vi "Version_4.9_8_on-chip_valves_for25ulSyringe_withModfied_Plunging.vi"() -> ()   [LabVIEW 2020] (continued)
                                n1270 = call "GoToAbsolutePosition(SubVI).vi"("Absolute Volume Position in Syringe (in ul)"=0.0 ("Volume to be Dispensed"), "Volume of Syringe"=w1733, "Resolution of Pumping"=w1732, "Flow Rate (ul/min)"=w1724, "VISA Refnum in"=w1734) -> ()  [unwired: 6 in, 1 out]
                                n1271 = local read "VISA Refnum in\nfor Valve"() -> (w1726:refnum<visa-resource-name>)
                                n1272 = local read "External Valve \nOPEN"() -> (w1725:string)
                                n1273 = local write "Valve V2 Open"(TRUE ("Valve V2 Open")) -> ()
                                n1274 = local write "Valve V1 Open"(FALSE ("Valve V1 Open")) -> ()
                                n1275 = local write "Valve V4 Open"(FALSE ("Valve V4 Open")) -> ()
                                n1276 = local write "Valve V3 Open"(TRUE ("Valve V3 Open")) -> ()
                                n1277 = call "PortChanger_Valve (SubVI).vi"("Port Number"=w1725, "VISA Refnum in"=w1726) -> ()  [unwired: 10 in]
                                }
                                frame #5 {
                                n1278 = local read "VISA Refnum in\nfor Pump"() -> (w1735:refnum<visa-resource-name>)
                                n1279 = call "ProcessCompletionWaiter (SubVI).vi"("VISA Refnum in"=w1735) -> ()  [unwired: 11 in]
                                }
                                frame #6 {
                                # "Change the port back to Buffer-C1"
                                n1280 = local read "VISA Refnum in\nfor Pump"() -> (w1737:refnum<visa-resource-name>)
                                n1281 = local read "Port for \nC1-Equilibriation"() -> (w1736:string)
                                n1282 = call "PortChanger (SubVI).vi"("Port Number"=w1736, "VISA Refnum in"=w1737) -> ()  [unwired: 10 in]
                                }
                                frame #7 {
                                n1283 = local read "VISA Refnum in\nfor Pump"() -> (w1738:refnum<visa-resource-name>)
                                n1284 = call "ProcessCompletionWaiter (SubVI).vi"("VISA Refnum in"=w1738) -> ()  [unwired: 11 in]
                                }
                              }
                            }
                          }
                          frame #4 {
                            # "Washes the SEC column"
                            n1285 = local read "Apparent Volume\nof Syringe"() -> (w1741:dbl)
                            n1286 = local read "c"() -> (w1742:dbl)
                            n1287 = Quotient & Remainder(x=w1742, y=w1741) -> (x-y*floor(x/y)=w1740:dbl, floor(x/y)=w1739:dbl)
                            n1288 = for {
                              N: w1739 -> [_]
                              n1289 = stacked-sequence {
                                frame #0 {
                                n1290 = local read "Buffer-A2 Pumping\nResolution"() -> (w1745:T2)
                                n1291 = local read "VISA Refnum in\nfor Pump"() -> (w1747:refnum<visa-resource-name>)
                                n1292 = local read "Apparent Volume\nof Syringe"() -> (w1743:dbl)
                                n1293 = local read "Volume of Syringe"() -> (w1746:dbl)
                                n1294 = call "RPickUp(SubVI).vi"("Volume to be picked up"=w1743, "Volume of Syringe"=w1746, "Resolution of PickUP"=w1745, "PickUp Flow Rate (ul/min)"=150.0, "VISA Refnum in"=w1747) -> ()  [unwired: 6 in, 1 out]
                                }
                                frame #1 {
                                n1295 = local read "Stopper that ends \nthe main loops"() -> (w1748:bool)
                                n1296 = local read "VISA Refnum in\nfor Pump"() -> (w1749:refnum<visa-resource-name>)
                                n1297 = case shown="True" w1748 {
                                frame False {
                                }
                                frame True {
                                n1298 = local read "VISA Refnum in\nfor Pump"() -> (w1750:refnum<visa-resource-name>)
                                n1299 = call "HardStopCurrentProcess (SubVI).vi"("VISA Refnum in"=w1750) -> ()  [unwired: 11 in]
                                }
                                }
                                n1300 = call "ProcessCompletionWaiter (SubVI).vi"("VISA Refnum in"=w1749) -> ()  [unwired: 11 in]
                                }
                                frame #2 {
                                # "Switch to Port-10"
                                # "Port-10 of the pump is conncted to column-2 of chip"
                                n1301 = local read "VISA Refnum in\nfor Pump"() -> (w1752:refnum<visa-resource-name>)
                                n1302 = call "PortChanger (SubVI).vi"("Port Number"="10", "VISA Refnum in"=w1752) -> ()  [unwired: 10 in]
                                }
                                frame #3 {
                                n1303 = local read "Stopper that ends \nthe main loops"() -> (w1753:bool)
                                n1304 = local read "VISA Refnum in\nfor Pump"() -> (w1754:refnum<visa-resource-name>)
                                n1305 = case shown="True" w1753 {
                                frame False {
                                }
                                frame True {
                                n1306 = local read "VISA Refnum in\nfor Pump"() -> (w1755:refnum<visa-resource-name>)
                                n1307 = call "HardStopCurrentProcess (SubVI).vi"("VISA Refnum in"=w1755) -> ()  [unwired: 11 in]
                                }
                                }
                                n1308 = call "ProcessCompletionWaiter (SubVI).vi"("VISA Refnum in"=w1754) -> ()  [unwired: 11 in]
                                }
                                frame #4 {
                                # "Keeps the AMF valve after column-1 open and valve after column-2 closed"
                                n1309 = local read "Buffer-A2 Pumping\nResolution"() -> (w1767:T2)
                                n1310 = local read "VISA Refnum in\nfor Pump"() -> (w1769:refnum<visa-resource-name>)
                                n1311 = local read "f"() -> (w1759:dbl)
                                n1312 = local write "Valve V3 Open"(FALSE ("Valve V3 Open")) -> ()
                                n1313 = local write "Valve V2 Open"(FALSE ("Valve V2 Open")) -> ()
                                n1314 = local write "Valve V4 Open"(TRUE ("Valve V4 Open")) -> ()
                                n1315 = local write "Valve V1 Open"(FALSE ("Valve V1 Open")) -> ()
                                n1316 = local read "Volume of Syringe"() -> (w1768:dbl)
                                n1317 = call "GoToAbsolutePosition(SubVI).vi"("Absolute Volume Position in Syringe (in ul)"=0.0 ("Volume to be Dispensed"), "Volume of Syringe"=w1768, "Resolution of Pumping"=w1767, "Flow Rate (ul/min)"=w1759, "VISA Refnum in"=w1769) -> ()  [unwired: 6 in, 1 out]
                                n1318 = local read "VISA Refnum in\nfor Valve"() -> (w1764:refnum<visa-resource-name>)
                                n1319 = local read "External Valve \nCLOSED"() -> (w1760:string)
                                n1320 = local write "Valve V5 Open"(TRUE ("Valve V5 Open")) -> ()
                                n1321 = local write "Valve V6 Open"(FALSE ("Valve V6 Open")) -> ()
                                n1322 = local write "Valve V7 Open"(TRUE ("Valve V7 Open")) -> ()
                                n1323 = call "PortChanger_Valve (SubVI).vi"("Port Number"=w1760, "VISA Refnum in"=w1764) -> ()  [unwired: 10 in]
                                }
                                frame #5 {
                                n1324 = local read "VISA Refnum in\nfor Pump"() -> (w1770:refnum<visa-resource-name>)
                                n1325 = call "ProcessCompletionWaiter (SubVI).vi"("VISA Refnum in"=w1770) -> ()  [unwired: 11 in]
                                }
                                frame #6 {
                                # "Change the port back to Buffer-C1"
                                n1326 = local read "VISA Refnum in\nfor Pump"() -> (w1772:refnum<visa-resource-name>)
                                n1327 = local read "Port for \nC1-Equilibriation"() -> (w1771:string)
                                n1328 = call "PortChanger (SubVI).vi"("Port Number"=w1771, "VISA Refnum in"=w1772) -> ()  [unwired: 10 in]
                                }
                                frame #7 {
                                n1329 = local read "VISA Refnum in\nfor Pump"() -> (w1773:refnum<visa-resource-name>)
                                n1330 = call "ProcessCompletionWaiter (SubVI).vi"("VISA Refnum in"=w1773) -> ()  [unwired: 11 in]
                                }
                              }
                            }
                            n1331 = local write "Reminder of the \nVolume to be \nPumped"(w1740) -> ()
                          }
                          frame #5 {
                            # "Washes the SEC column"
                            n1332 = stacked-sequence {
                              frame #0 {
                                n1333 = local read "Buffer-A2 Pumping\nResolution"() -> (w1776:T2)
                                n1334 = local read "VISA Refnum in\nfor Pump"() -> (w1778:refnum<visa-resource-name>)
                                n1335 = local read "Reminder of the \nVolume to be \nPumped"() -> (w1774:dbl)
                                n1336 = local read "Volume of Syringe"() -> (w1777:dbl)
                                n1337 = call "RPickUp(SubVI).vi"("Volume to be picked up"=w1774, "Volume of Syringe"=w1777, "Resolution of PickUP"=w1776, "PickUp Flow Rate (ul/min)"=150.0, "VISA Refnum in"=w1778) -> ()  [unwired: 6 in, 1 out]
                              }
                              frame #1 {
                                n1338 = local read "Stopper that ends \nthe main loops"() -> (w1779:bool)
                                n1339 = local read "VISA Refnum in\nfor Pump"() -> (w1780:refnum<visa-resource-name>)
                                n1340 = case shown="True" w1779 {
                                frame False {
                                }
                                frame True {
                                n1341 = local read "VISA Refnum in\nfor Pump"() -> (w1781:refnum<visa-resource-name>)
                                n1342 = call "HardStopCurrentProcess (SubVI).vi"("VISA Refnum in"=w1781) -> ()  [unwired: 11 in]
                                }
                                }
                                n1343 = call "ProcessCompletionWaiter (SubVI).vi"("VISA Refnum in"=w1780) -> ()  [unwired: 11 in]
                              }
                              frame #2 {
                                # "Switch to Port-10"
                                # "Port-10 of the pump is conncted to column-2 of chip"
                                n1344 = local read "VISA Refnum in\nfor Pump"() -> (w1783:refnum<visa-resource-name>)
                                n1345 = call "PortChanger (SubVI).vi"("Port Number"="10", "VISA Refnum in"=w1783) -> ()  [unwired: 10 in]
                              }
                              frame #3 {
                                n1346 = local read "Stopper that ends \nthe main loops"() -> (w1784:bool)
                                n1347 = local read "VISA Refnum in\nfor Pump"() -> (w1785:refnum<visa-resource-name>)
                                n1348 = case shown="True" w1784 {
                                frame False {
                                }
                                frame True {
                                n1349 = local read "VISA Refnum in\nfor Pump"() -> (w1786:refnum<visa-resource-name>)
                                n1350 = call "HardStopCurrentProcess (SubVI).vi"("VISA Refnum in"=w1786) -> ()  [unwired: 11 in]
                                }
                                }
                                n1351 = call "ProcessCompletionWaiter (SubVI).vi"("VISA Refnum in"=w1785) -> ()  [unwired: 11 in]
                              }
                              frame #4 {
                                n1352 = local read "Buffer-A2 Pumping\nResolution"() -> (w1798:T2)
                                n1353 = local read "VISA Refnum in\nfor Pump"() -> (w1800:refnum<visa-resource-name>)
                                n1354 = local read "f"() -> (w1790:dbl)
                                n1355 = local read "Volume of Syringe"() -> (w1799:dbl)
                                n1356 = call "GoToAbsolutePosition(SubVI).vi"("Absolute Volume Position in Syringe (in ul)"=0.0 ("Volume to be Dispensed"), "Volume of Syringe"=w1799, "Resolution of Pumping"=w1798, "Flow Rate (ul/min)"=w1790, "VISA Refnum in"=w1800) -> ()  [unwired: 6 in, 1 out]
                                n1357 = local write "Valve V3 Open"(FALSE ("Valve V3 Open")) -> ()
                                n1358 = local write "Valve V2 Open"(FALSE ("Valve V2 Open")) -> ()
                                n1359 = local write "Valve V1 Open"(FALSE ("Valve V1 Open")) -> ()
                                n1360 = local write "Valve V4 Open"(TRUE ("Valve V4 Open")) -> ()
                                n1361 = local read "VISA Refnum in\nfor Valve"() -> (w1795:refnum<visa-resource-name>)
                                n1362 = local read "External Valve \nCLOSED"() -> (w1791:string)
                                n1363 = local write "Valve V6 Open"(TRUE ("Valve V6 Open")) -> ()
                                n1364 = local write "Valve V5 Open"(TRUE ("Valve V5 Open")) -> ()
                                n1365 = local write "Valve V7 Open"(TRUE ("Valve V7 Open")) -> ()
                                n1366 = call "PortChanger_Valve (SubVI).vi"("Port Number"=w1791, "VISA Refnum in"=w1795) -> ()  [unwired: 10 in]
                              }
                              frame #5 {
                                n1367 = local read "VISA Refnum in\nfor Pump"() -> (w1801:refnum<visa-resource-name>)
                                n1368 = call "ProcessCompletionWaiter (SubVI).vi"("VISA Refnum in"=w1801) -> ()  [unwired: 11 in]
                              }
                            }
                          }
                        }
                        n1369 = local write "Washing Column-1"(FALSE ("Washing Column-1")) -> ()
                        n1370 = local write "Washing Column-2"(TRUE ("Washing Column-2")) -> ()
                      }
                      frame #4 {
                        # "Elute Column-1, Divert Sample into Column-2, Elute column-2 and Divert the sample onto Grid"
                        n1371 = stacked-sequence {
                          frame #0 {
                            # "Switch to Port-7"
                            # "Port-7 of pump is connected to Buffer-B"
                            n1372 = local write "Washing Column-2"(FALSE ("Washing Column-2")) -> ()
                            n1373 = local read "VISA Refnum in\nfor Pump"() -> (w1806:refnum<visa-resource-name>)
                            n1374 = local read "Port for \nB-Elution"() -> (w1804:string)
                            n1375 = local write "Affinity Elution On"(TRUE ("Affinity Elution On")) -> ()
                            n1376 = call "PortChanger (SubVI).vi"("Port Number"=w1804, "VISA Refnum in"=w1806) -> ()  [unwired: 10 in]
                            n1377 = local write "Elution of Column-1"(TRUE ("Elution of Column-1")) -> ()
                          }
                          frame #1 {
                            n1378 = local read "VISA Refnum in\nfor Pump"() -> (w1807:refnum<visa-resource-name>)
                            n1379 = call "ProcessCompletionWaiter (SubVI).vi"("VISA Refnum in"=w1807) -> ()  [unwired: 11 in]
                          }
                          frame #2 {
                            # "If Yes, it will clean the elution buffer from port-5 tubing a bit more"
                            n1380 = local read "Clean the \nBuffer-B tubing"() -> (w1808:bool)
                            n1381 = case shown="True" w1808 {
                              frame False {
                                n1382 = stacked-sequence {
                                frame #0 {
                                n1383 = local read "Buffer-B Pumping\nResolution"() -> (w1811:T2)
                                n1384 = local read "VISA Refnum in\nfor Pump"() -> (w1813:refnum<visa-resource-name>)
                                n1385 = local read "V-S"() -> (w1810:dbl)
                                n1386 = local read "Volume of Syringe"() -> (w1812:dbl)
                                n1387 = call "RPickUp(SubVI).vi"("Volume to be picked up"=w1810, "Volume of Syringe"=w1812, "Resolution of PickUP"=w1811, "PickUp Flow Rate (ul/min)"=150.0, "VISA Refnum in"=w1813) -> ()  [unwired: 6 in, 1 out]
                                }
                                frame #1 {
                                n1388 = local read "Stopper that ends \nthe main loops"() -> (w1814:bool)
                                n1389 = local read "VISA Refnum in\nfor Pump"() -> (w1815:refnum<visa-resource-name>)
                                n1390 = case shown="True" w1814 {
                                frame False {
                                }
                                frame True {
                                n1391 = local read "VISA Refnum in\nfor Pump"() -> (w1816:refnum<visa-resource-name>)
                                n1392 = call "HardStopCurrentProcess (SubVI).vi"("VISA Refnum in"=w1816) -> ()  [unwired: 11 in]
                                }
                                }
                                n1393 = call "ProcessCompletionWaiter (SubVI).vi"("VISA Refnum in"=w1815) -> ()  [unwired: 11 in]
                                }
                                frame #2 {
                                n1394 = local read "VISA Refnum in\nfor Pump"() -> (w1818:refnum<visa-resource-name>)
                                n1395 = call "PortChanger (SubVI).vi"("Port Number"="1", "VISA Refnum in"=w1818) -> ()  [unwired: 10 in]
                                }
                                frame #3 {
                                n1396 = local read "Stopper that ends \nthe main loops"() -> (w1819:bool)
                                n1397 = local read "VISA Refnum in\nfor Pump"() -> (w1820:refnum<visa-resource-name>)
                                n1398 = case shown="True" w1819 {
                                frame False {
                                }
                                frame True {
                                n1399 = local read "VISA Refnum in\nfor Pump"() -> (w1821:refnum<visa-resource-name>)
                                n1400 = call "HardStopCurrentProcess (SubVI).vi"("VISA Refnum in"=w1821) -> ()  [unwired: 11 in]
                                }
                                }
                                n1401 = call "ProcessCompletionWaiter (SubVI).vi"("VISA Refnum in"=w1820) -> ()  [unwired: 11 in]
                                }
                                frame #4 {
                                n1402 = local read "VISA Refnum in\nfor Pump"() -> (w1826:refnum<visa-resource-name>)
                                n1403 = local read "Volume of Syringe"() -> (w1823:dbl)
                                n1404 = call "GoToAbsolutePosition(SubVI).vi"("Absolute Volume Position in Syringe (in ul)"=0.0, "Volume of Syringe"=w1823, "Resolution of Pumping"=T2."Standard Pumping", "Flow Rate (ul/min)"=150.0, "VISA Refnum in"=w1826) -> ()  [unwired: 6 in, 1 out]
                                }
                                frame #5 {
                                n1405 = local read "Stopper that ends \nthe main loops"() -> (w1827:bool)
                                n1406 = local read "VISA Refnum in\nfor Pump"() -> (w1828:refnum<visa-resource-name>)
                                n1407 = case shown="True" w1827 {
                                frame False {
                                }
                                frame True {
                                n1408 = local read "VISA Refnum in\nfor Pump"() -> (w1829:refnum<visa-resource-name>)
                                n1409 = call "HardStopCurrentProcess (SubVI).vi"("VISA Refnum in"=w1829) -> ()  [unwired: 11 in]
                                }
                                }
                                n1410 = call "ProcessCompletionWaiter (SubVI).vi"("VISA Refnum in"=w1828) -> ()  [unwired: 11 in]
                                }
                                }
                              }
                              frame True {
                                n1411 = for {
                                N: 2 -> [_]
                                n1412 = stacked-sequence {
                                frame #0 {
                                n1413 = local read "Buffer-B Pumping\nResolution"() -> (w1833:T2)
                                n1414 = local read "VISA Refnum in\nfor Pump"() -> (w1835:refnum<visa-resource-name>)
                                n1415 = local read "Apparent Volume\nof Syringe"() -> (w1832:dbl)
                                n1416 = local read "Volume of Syringe"() -> (w1834:dbl)
                                n1417 = call "RPickUp(SubVI).vi"("Volume to be picked up"=w1832, "Volume of Syringe"=w1834, "Resolution of PickUP"=w1833, "PickUp Flow Rate (ul/min)"=150.0, "VISA Refnum in"=w1835) -> ()  [unwired: 6 in, 1 out]
                                }
                                frame #1 {
                                n1418 = local read "Stopper that ends \nthe main loops"() -> (w1836:bool)
                                n1419 = local read "VISA Refnum in\nfor Pump"() -> (w1837:refnum<visa-resource-name>)
                                n1420 = case shown="True" w1836 {
                                frame False {
                                }
                                frame True {
                                n1421 = local read "VISA Refnum in\nfor Pump"() -> (w1838:refnum<visa-resource-name>)
                                n1422 = call "HardStopCurrentProcess (SubVI).vi"("VISA Refnum in"=w1838) -> ()  [unwired: 11 in]
                                }
                                }
                                n1423 = call "ProcessCompletionWaiter (SubVI).vi"("VISA Refnum in"=w1837) -> ()  [unwired: 11 in]
                                }
                                frame #2 {
                                n1424 = local read "VISA Refnum in\nfor Pump"() -> (w1840:refnum<visa-resource-name>)
                                n1425 = call "PortChanger (SubVI).vi"("Port Number"="1", "VISA Refnum in"=w1840) -> ()  [unwired: 10 in]
                                }
                                frame #3 {
                                n1426 = local read "Stopper that ends \nthe main loops"() -> (w1841:bool)
                                n1427 = local read "VISA Refnum in\nfor Pump"() -> (w1842:refnum<visa-resource-name>)
                                n1428 = case shown="True" w1841 {
                                frame False {
                                }
                                frame True {
                                n1429 = local read "VISA Refnum in\nfor Pump"() -> (w1843:refnum<visa-resource-name>)
                                n1430 = call "HardStopCurrentProcess (SubVI).vi"("VISA Refnum in"=w1843) -> ()  [unwired: 11 in]
                                }
                                }
                                n1431 = call "ProcessCompletionWaiter (SubVI).vi"("VISA Refnum in"=w1842) -> ()  [unwired: 11 in]
                                }
                                frame #4 {
                                n1432 = local read "VISA Refnum in\nfor Pump"() -> (w1848:refnum<visa-resource-name>)
                                n1433 = local read "Volume of Syringe"() -> (w1845:dbl)
                                n1434 = call "GoToAbsolutePosition(SubVI).vi"("Absolute Volume Position in Syringe (in ul)"=0.0, "Volume of Syringe"=w1845, "Resolution of Pumping"=T2."Standard Pumping", "Flow Rate (ul/min)"=150.0, "VISA Refnum in"=w1848) -> ()  [unwired: 6 in, 1 out]
                                }
                                frame #5 {
                                n1435 = local read "Stopper that ends \nthe main loops"() -> (w1849:bool)
                                n1436 = local read "VISA Refnum in\nfor Pump"() -> (w1850:refnum<visa-resource-name>)
                                n1437 = case shown="True" w1849 {
                                frame False {
                                }
                                frame True {
                                n1438 = local read "VISA Refnum in\nfor Pump"() -> (w1851:refnum<visa-resource-name>)
                                n1439 = call "HardStopCurrentProcess (SubVI).vi"("VISA Refnum in"=w1851) -> ()  [unwired: 11 in]
                                }
                                }
                                n1440 = call "ProcessCompletionWaiter (SubVI).vi"("VISA Refnum in"=w1850) -> ()  [unwired: 11 in]
                                }
                                }
                                }
                              }
                            }
                          }
                          frame #3 {
                            n1441 = local read "VISA Refnum in\nfor Pump"() -> (w1853:refnum<visa-resource-name>)
                            n1442 = local read "Port for \nB-Elution"() -> (w1852:string)
                            n1443 = call "PortChanger (SubVI).vi"("Port Number"=w1852, "VISA Refnum in"=w1853) -> ()  [unwired: 10 in]
                          }
                          frame #4 {
                            n1444 = local read "VISA Refnum in\nfor Pump"() -> (w1854:refnum<visa-resource-name>)
                            n1445 = call "ProcessCompletionWaiter (SubVI).vi"("VISA Refnum in"=w1854) -> ()  [unwired: 11 in]
                          }
                          frame #5 {
                            n1446 = local read "Buffer-B PickUp \nFlow Rate (ul/min)"() -> (w1857:dbl)
                            n1447 = local read "Buffer-B Pumping\nResolution"() -> (w1856:T2)
                            n1448 = local read "VISA Refnum in\nfor Pump"() -> (w1859:refnum<visa-resource-name>)
                            n1449 = local read "Buffer-B Volume \nto be  Pumped"() -> (w1855:dbl)
                            n1450 = local read "Volume of Syringe"() -> (w1858:dbl)
                            n1451 = call "RPickUp(SubVI).vi"("Volume to be picked up"=w1855, "Volume of Syringe"=w1858, "Resolution of PickUP"=w1856, "PickUp Flow Rate (ul/min)"=w1857, "VISA Refnum in"=w1859) -> ()  [unwired: 6 in, 1 out]
                          }
                          frame #6 {
                            n1452 = local read "Stopper that ends \nthe main loops"() -> (w1860:bool)
                            n1453 = local read "VISA Refnum in\nfor Pump"() -> (w1861:refnum<visa-resource-name>)
                            n1454 = case shown="True" w1860 {
                              frame False {
                              }
                              frame True {
                                n1455 = local read "VISA Refnum in\nfor Pump"() -> (w1862:refnum<visa-resource-name>)
                                n1456 = call "HardStopCurrentProcess (SubVI).vi"("VISA Refnum in"=w1862) -> ()  [unwired: 11 in]
                              }
                            }
                            n1457 = call "ProcessCompletionWaiter (SubVI).vi"("VISA Refnum in"=w1861) -> ()  [unwired: 11 in]
                          }
                          frame #7 {
                            # "Reads the initial Plunger Position for computing the volume dispensed"
                            n1458 = local read "VISA Refnum in\nfor Pump"() -> (w1864:refnum<visa-resource-name>)
                            n1459 = call "AbsolutePlungerPosition (SubVI).vi"("VISA Refnum in"=w1864) -> ("Plunger Position"=w1863:i32)  [unwired: 10 in]
                            n1460 = local write "Initial Plunger Position"(w1863) -> ()
                          }
                          frame #8 {
                            # "Switch to Port-2"
                            # "Port-2 of the pump is conncted to column-1 of chip"
                            n1461 = local read "VISA Refnum in\nfor Pump"() -> (w1866:refnum<visa-resource-name>)
                            n1462 = call "PortChanger (SubVI).vi"("Port Number"="2", "VISA Refnum in"=w1866) -> ()  [unwired: 10 in]
                          }
                          frame #9 {
                            n1463 = local read "Stopper that ends \nthe main loops"() -> (w1867:bool)
                            n1464 = local read "VISA Refnum in\nfor Pump"() -> (w1868:refnum<visa-resource-name>)
                            n1465 = case shown="True" w1867 {
                              frame False {
                              }
                              frame True {
                                n1466 = local read "VISA Refnum in\nfor Pump"() -> (w1869:refnum<visa-resource-name>)
                                n1467 = call "HardStopCurrentProcess (SubVI).vi"("VISA Refnum in"=w1869) -> ()  [unwired: 11 in]
                              }
                            }
                            n1468 = call "ProcessCompletionWaiter (SubVI).vi"("VISA Refnum in"=w1868) -> ()  [unwired: 11 in]
                          }
                          frame #10 {
                            # "Keeps the AMF valve after column-1 open and valve after column-2 closed"
                            n1469 = local read "VISA Refnum in\nfor Valve"() -> (w1874:refnum<visa-resource-name>)
                            n1470 = local read "External Valve \nOPEN"() -> (w1873:string)
                            n1471 = call "PortChanger_Valve (SubVI).vi"("Port Number"=w1873, "VISA Refnum in"=w1874) -> ()  [unwired: 10 in]
                            n1472 = local write "Valve V1 Open"(TRUE ("Valve V1 Open")) -> ()
                            n1473 = local write "Valve V2 Open"(TRUE ("Valve V2 Open")) -> ()
                            n1474 = local write "Valve V3 Open"(FALSE ("Valve V3 Open")) -> ()
                            n1475 = local write "Valve V4 Open"(FALSE ("Valve V4 Open")) -> ()
                            n1476 = local write "Valve V6 Open"(FALSE ("Valve V6 Open")) -> ()
                            n1477 = local write "Valve V5 Open"(FALSE ("Valve V5 Open")) -> ()
                            n1478 = local write "Valve V7 Open"(FALSE ("Valve V7 Open")) -> ()
                          }
                          frame #11 {
                            n1479 = local read "Buffer-B Dispense\nFlow Rate (ul/min)"() -> (w1884:dbl)
                            n1480 = local read "Buffer-B Pumping\nResolution"() -> (w1883:T2)
                            n1481 = local read "Initial Plunger Position"() -> (w1880:dbl)
                            n1482 = local read "VISA Refnum in\nfor Pump"() -> (w1886:refnum<visa-resource-name>)
                            n1483 = local read "Volume of Syringe"() -> (w1885:dbl)
                            n1484 = call "GoToAbsolutePosition(SubVI).vi"("Absolute Volume Position in Syringe (in ul)"=0.0 ("Volume to be Dispensed"), "Volume of Syringe"=w1885, "Resolution of Pumping"=w1883, "Flow Rate (ul/min)"=w1884, "VISA Refnum in"=w1886) -> ()  [unwired: 6 in, 1 out]
                            n1485 = local write "Pause Data Collection"(FALSE ("Pause Data Collection")) -> ()
                            n1486 = local write "Vol_now"(0.0 ("Vol_now")) -> ()
                            n1487 = local write "Position\nNow"(w1880) -> ()
                          }
                          frame #12 {
                            n1488 = while {
                              stop <- w1893 stop-if-true
                              n1489 = event shown="[1] Timeout" {
                                selector: _ -> [_ _]
                                dyn-events: _ -> [_ _]
                                timeout: 100 -> [_ _]
                                event "Pause Elution\nValue": Value Change {
                                n1490 = event-data() -> ()  [unwired: 1 in, 6 out]
                                n1491 = stacked-sequence {
                                frame #0 {
                                n1492 = local read "Pause Elution"() -> (w1895:bool)
                                n1493 = case shown="False" w1895 {
                                frame False {
                                n1494 = local write "Pause Elution"(TRUE ("Pause Elution")) -> ()
                                }
                                frame True {
                                n1495 = local write "Pause Elution"(FALSE ("Pause Elution")) -> ()
                                }
                                }
                                }
                                frame #1 {
                                n1496 = local read "Pause Elution"() -> (w1898:bool)
                                n1497 = case shown="False" w1898 {
                                frame False {
                                n1498 = local read "Buffer-B Dispense\nFlow Rate (ul/min)"() -> (w1903:dbl)
                                n1499 = local read "VISA Refnum in\nfor Pump"() -> (w1904:refnum<visa-resource-name>)
                                n1500 = local read "Buffer-B Pumping\nResolution"() -> (w1900:T2)
                                n1501 = local read "Volume of Syringe"() -> (w1901:dbl)
                                n1502 = call "GoToAbsolutePosition(SubVI).vi"("Absolute Volume Position in Syringe (in ul)"=0.0, "Volume of Syringe"=w1901, "Resolution of Pumping"=w1900, "Flow Rate (ul/min)"=w1903, "VISA Refnum in"=w1904) -> ()  [unwired: 6 in, 1 out]
                                n1503 = local write "Pause Data Collection"(FALSE ("Pause Data Collection")) -> ()
                                }
                                frame True {
                                n1504 = local read "VISA Refnum in\nfor Pump"() -> (w1906:refnum<visa-resource-name>)
                                n1505 = local write "Pause Data Collection"(TRUE ("Pause Data Collection")) -> ()
                                n1506 = call "HardStopCurrentProcess (SubVI).vi"("VISA Refnum in"=w1906) -> ()  [unwired: 11 in]
                                }
                                }
                                }
                                }
                                }
                                event Timeout {
                                n1507 = event-data() -> ()  [unwired: 1 in, 3 out]
                                }
                              }
                              n1508 = local read "Stopper that ends \nthe main loops"() -> (w1892:bool)
                              n1509 = local read "Divert Sample \ninto Column-2"() -> (w1891:bool)
                              n1510 = Or(x=w1891, y=w1892) -> (x .or. y?=w1893:bool)
                            }
                            n1511 = local read "Buffer-B Pumping\nResolution"() -> (w1889:T2)
                            n1512 = local read "VISA Refnum in\nfor Pump"() -> (w1890:refnum<visa-resource-name>)
                            n1513 = local read "Volume of Syringe"() -> (w1888:dbl)
                            n1514 = while {
                              tunnel: w1890 -> [w1915]
                              tunnel: w1889 -> [w1914]
                              tunnel: w1888 -> [w1913]
                              stop <- w1909 stop-if-true
                              n1515 = local read "Position\nNow"() -> (w1907:dbl)
                              n1516 = local read "Pause Elution"() -> (w1908:bool)
                              n1517 = case shown="True" w1908 {
                                tunnel: w1907 -> [w1919 _]
                                tunnel: w1915 -> [w1918 w1961]
                                tunnel: w1914 -> [w1917 _]
                                tunnel: w1913 -> [w1916 _]
                                frame False {
                                n1518 = stacked-sequence {
                                tunnel: w1919 -> [_ w1925]
                                tunnel: w1918 -> [_ w1924]
                                tunnel: w1917 -> [_ w1923]
                                tunnel: w1916 -> [_ w1922]
                                frame #0 {
                                n1519 = Wait (ms)(milliseconds to wait=u32 3000) -> ()  [unwired: 1 out]
                                n1520 = local write "Signal"(TRUE ("Signal")) -> ()
                                }
                                frame #1 {
                                n1521 = while {
                                tunnel: w1925 -> [w1937]
                                tunnel: w1924 -> [w1936]
                                tunnel: w1923 -> [w1935]
                                tunnel: w1922 -> [w1934]
                                stop <- w1929 stop-if-true
                                n1522 = stacked-sequence {
                                tunnel: w1937 -> [_ w1944]
                                tunnel: w1936 -> [_ w1943]
                                tunnel: w1935 -> [_ w1942]
                                tunnel: w1934 -> [_ w1941]
                                frame #0 {
                                n1523 = Wait (ms)(milliseconds to wait=u32 500) -> ()  [unwired: 1 out]
                                }
                                frame #1 {
                                n1524 = call "AbsolutePlungerPosition (SubVI).vi"("VISA Refnum in"=w1943) -> ("Plunger Position"=w1940:i32)  [unwired: 10 in]
                                n1525 = case shown="\"High Resolution Pumping\"" w1942 {
                                tunnel: w1944 -> [w1949 w1958]
                                tunnel: w1940 -> [w1950 w1957]
                                tunnel: [w1948 w1955] -> w1939
                                tunnel: w1941 -> [w1947 w1956]
                                frame "Standard Pumping", Default {
                                n1526 = Subtract(x=w1949, y=w1950) -> (x-y=w1946:dbl)
                                n1527 = Absolute Value(x=w1946) -> (abs(x)=w1945:dbl)
                                n1528 = Multiply(x=w1945, y=w1947) -> (x*y=w1952:dbl)
                                n1529 = Divide(x=w1952, y=3000.0) -> (x/y=w1948:dbl)
                                }
                                frame "High Resolution Pumping" {
                                n1530 = Subtract(x=w1958, y=w1957) -> (x-y=w1954:dbl)
                                n1531 = Absolute Value(x=w1954) -> (abs(x)=w1953:dbl)
                                n1532 = Multiply(x=w1953, y=w1956) -> (x*y=w1960:dbl)
                                n1533 = Divide(x=w1960, y=24000.0) -> (x/y=w1955:dbl)
                                }
                                }
                                n1534 = local write "Volume being Injected \nin this process"(w1939) -> ()
                                }
                                }
                                n1535 = local read "Volume being Injected \nin this process"() -> (w1927:dbl)
                                n1536 = local read "Affinity Elution \nGraph Min CutOff"() -> (w1926:dbl)
                                n1537 = local read "Stopper that ends \nthe main loops"() -> (w1932:bool)
                                n1538 = local read "Divert Sample \ninto Column-2"() -> (w1933:bool)
                                n1539 = Greater Or Equal?(x=w1927, y=w1926) -> (x >= y?=w1928:bool)
                                n1540 = Or(x=w1933, y=w1932) -> (x .or. y?=w1930:bool)
                                n1541 = local read "Pause Elution"() -> (w1931:bool)
                                n1542 = local write "Affinity Elution \nis Approaching"(w1928) -> ()
                                n1543 = Or(x=w1931, y=w1930) -> (x .or. y?=w1929:bool)
                                }
                                }
                                }
                                }
                                frame True {
                                n1544 = stacked-sequence {
                                tunnel: w1961 -> [_ w1964 _]
                                frame #0 {
                                n1545 = Wait (ms)(milliseconds to wait=u32 2000) -> ()  [unwired: 1 out]
                                }
                                frame #1 {
                                n1546 = local read "Signal"() -> (w1963:bool)
                                n1547 = case shown="True" w1963 {
                                tunnel: w1964 -> [_ w1970]
                                frame False {
                                }
                                frame True {
                                n1548 = local read "Volume being Injected \nin this process"() -> (w1968:dbl)
                                n1549 = local read "Net Elution \nVolume"() -> (w1967:dbl)
                                n1550 = local write "Signal"(FALSE ("Signal")) -> ()
                                n1551 = Add(x=w1968, y=w1967) -> (x+y=w1966:dbl)
                                n1552 = call "AbsolutePlungerPosition (SubVI).vi"("VISA Refnum in"=w1970) -> ("Plunger Position"=w1969:i32)  [unwired: 10 in]
                                n1553 = local write "Net Elution \nVolume"(w1966) -> ()
                                n1554 = local write "Position\nNow"(w1969) -> ()
                                }
                                }
                                }
                                frame #2 {
                                n1555 = local write "Volume being Injected \nin this process"(0.0 ("Volume being Injected \nin this process")) -> ()
                                }
                                }
                                }
                              }
                              n1556 = local read "Stopper that ends \nthe main loops"() -> (w1911:bool)
                              n1557 = local read "Divert Sample \ninto Column-2"() -> (w1910:bool)
                              n1558 = Or(x=w1910, y=w1911) -> (x .or. y?=w1909:bool)
                              n1559 = Wait (ms)(milliseconds to wait=u32 300) -> ()  [unwired: 1 out]
                            }
                            n1560 = local read "Stopper that ends \nthe main loops"() -> (w1887:bool)
                            n1561 = case shown="True" w1887 {
                              frame False {
                              }
                              frame True {
                                n1562 = local read "VISA Refnum in\nfor Pump"() -> (w1972:refnum<visa-resource-name>)
                                n1563 = call "HardStopCurrentProcess (SubVI).vi"("VISA Refnum in"=w1972) -> ()  [unwired: 11 in]
                              }
                            }
                          }
                          frame #13 {
                            # "valve after column-1 is closed"
                            # "Keeps the on-chip Valve V1 and V3 after column-2 open"
                            # "Keeps the AMF valve after column-1 closed and valve after column-2 open"
                            n1564 = local read "VISA Refnum in\nfor Pump"() -> (w1985:refnum<visa-resource-name>)
                            n1565 = local read "Volume being Injected \nin this process"() -> (w1982:dbl)
                            n1566 = local write "Sample Volume Diverted\ninto Column-2"(0.0 ("Sample Volume Diverted\ninto Column-2")) -> ()
                            n1567 = call "AbsolutePlungerPosition (SubVI).vi"("VISA Refnum in"=w1985) -> ("Plunger Position"=w1984:i32)  [unwired: 10 in]
                            n1568 = local write "Position\nNow"(w1984) -> ()
                            n1569 = local write "Vol_previous"(0.0 ("Vol_diff")) -> ()
                            n1570 = local write "Vol_now"(w1982) -> ()
                            n1571 = local read "VISA Refnum in\nfor Valve"() -> (w1977:refnum<visa-resource-name>)
                            n1572 = local read "External Valve \nCLOSED"() -> (w1976:string)
                            n1573 = local write "Valve V1 Open"(TRUE ("Valve V1 Open")) -> ()
                            n1574 = local write "Valve V3 Open"(TRUE ("Valve V3 Open")) -> ()
                            n1575 = local write "Valve V2 Open"(FALSE ("Valve V2 Open")) -> ()
                            n1576 = local write "Valve V4 Open"(TRUE ("Valve V4 Open")) -> ()
                            n1577 = call "PortChanger_Valve (SubVI).vi"("Port Number"=w1976, "VISA Refnum in"=w1977) -> ()  [unwired: 10 in]
                            n1578 = local write "Valve V5 Open"(TRUE ("Valve V5 Open")) -> ()
                            n1579 = local write "Valve V6 Open"(FALSE ("Valve V6 Open")) -> ()
                            n1580 = local write "Valve V7 Open"(TRUE ("Valve V7 Open")) -> ()
                          }
                          frame #14 {
                            n1581 = local read "Divert Sample \ninto Column-2"() -> (w1987:bool)
                            n1582 = case shown="True" w1987 {
                              frame False {
                                n1583 = stacked-sequence {
                                frame #0 {
                                n1584 = local read "Buffer-B Pumping\nResolution"() -> (w1990:T2)
                                n1585 = local read "VISA Refnum in\nfor Pump"() -> (w1992:refnum<visa-resource-name>)
                                n1586 = local read "Initial Plunger Position"() -> (w1991:dbl)
                                n1587 = local read "Volume of Syringe"() -> (w1989:dbl)
                                n1588 = while {
                                tunnel: w1991 -> [w1998]
                                tunnel: w1992 -> [w1997]
                                tunnel: w1990 -> [w1996]
                                tunnel: w1989 -> [w1995]
                                stop <- w1993 stop-if-true
                                n1589 = Wait (ms)(milliseconds to wait=u32 100) -> ()  [unwired: 1 out]
                                n1590 = stacked-sequence {
                                tunnel: w1998 -> [w2004 _]
                                tunnel: w1997 -> [w2003 w2024]
                                tunnel: w1996 -> [w2002 _]
                                tunnel: w1995 -> [w2001 _]
                                tunnel: [_ w2022] -> w1993
                                frame #0 {
                                n1591 = call "AbsolutePlungerPosition (SubVI).vi"("VISA Refnum in"=w2003) -> ("Plunger Position"=w2000:i32)  [unwired: 10 in]
                                n1592 = case shown="\"Standard Pumping\", Default" w2002 {
                                tunnel: w2004 -> [w2009 w2018]
                                tunnel: w2000 -> [w2010 w2017]
                                tunnel: [w2008 w2015] -> w1999
                                tunnel: w2001 -> [w2007 w2016]
                                frame "Standard Pumping", Default {
                                n1593 = Subtract(x=w2009, y=w2010) -> (x-y=w2006:dbl)
                                n1594 = Absolute Value(x=w2006) -> (abs(x)=w2005:dbl)
                                n1595 = Multiply(x=w2005, y=w2007) -> (x*y=w2012:dbl)
                                n1596 = Divide(x=w2012, y=3000.0) -> (x/y=w2008:dbl)
                                }
                                frame "High Resolution Pumping" {
                                n1597 = Subtract(x=w2018, y=w2017) -> (x-y=w2014:dbl)
                                n1598 = Absolute Value(x=w2014) -> (abs(x)=w2013:dbl)
                                n1599 = Multiply(x=w2013, y=w2016) -> (x*y=w2020:dbl)
                                n1600 = Divide(x=w2020, y=24000.0) -> (x/y=w2015:dbl)
                                }
                                }
                                n1601 = local write "Volume being Injected \nin this process"(w1999) -> ()
                                }
                                frame #1 {
                                n1602 = local read "Stopper that ends \nthe main loops"() -> (w2021:bool)
                                n1603 = call "LSPOneStatus (SubVI).vi"("VISA Refnum in"=w2024) -> ("read buffer"=w2026:string)  [unwired: 10 in]
                                n1604 = call <vilib>:"Trim Whitespace.vi"("string"=w2026) -> ("trimmed string"=w2025:string)  [unwired: 1 in]
                                n1605 = Equal?(x=w2025, y="/0`\u0003") -> (x = y?=w2023:bool)
                                n1606 = Or(x=w2023, y=w2021) -> (x .or. y?=w2022:bool)
                                }
                                }
                                }
                                n1607 = local read "Stopper that ends \nthe main loops"() -> (w1988:bool)
                                n1608 = case shown="True" w1988 {
                                frame False {
                                }
                                frame True {
                                n1609 = local read "VISA Refnum in\nfor Pump"() -> (w2028:refnum<visa-resource-name>)
                                n1610 = call "HardStopCurrentProcess (SubVI).vi"("VISA Refnum in"=w2028) -> ()  [unwired: 11 in]
                                }
                                }
                                }
                                }
                              }
                              frame True {
                                n1611 = stacked-sequence {
                                frame #0 {
                                n1612 = local read "Buffer-B Pumping\nResolution"() -> (w2031:T2)
                                n1613 = local read "VISA Refnum in\nfor Pump"() -> (w2033:refnum<visa-resource-name>)
                                n1614 = local read "Volume of Syringe"() -> (w2030:dbl)
                                n1615 = local read "Position\nNow"() -> (w2032:dbl)
                                n1616 = while {
                                tunnel: w2032 -> [w2039]
                                tunnel: w2033 -> [w2038]
                                tunnel: w2031 -> [w2037]
                                tunnel: w2030 -> [w2036]
                                stop <- w2034 stop-if-true
                                n1617 = Wait (ms)(milliseconds to wait=u32 100) -> ()  [unwired: 1 out]
                                n1618 = stacked-sequence {
                                tunnel: w2039 -> [w2049 _ _]
                                tunnel: w2038 -> [w2048 _ w2075]
                                tunnel: w2037 -> [w2047 _ _]
                                tunnel: w2036 -> [w2046 _ _]
                                tunnel: [_ _ w2073] -> w2034
                                frame #0 {
                                n1619 = local read "Vol_previous"() -> (w2043:dbl)
                                n1620 = call "AbsolutePlungerPosition (SubVI).vi"("VISA Refnum in"=w2048) -> ("Plunger Position"=w2045:i32)  [unwired: 10 in]
                                n1621 = case shown="\"Standard Pumping\", Default" w2047 {
                                tunnel: w2049 -> [w2054 w2063]
                                tunnel: w2045 -> [w2055 w2062]
                                tunnel: [w2053 w2060] -> w2044
                                tunnel: w2046 -> [w2052 w2061]
                                frame "Standard Pumping", Default {
                                n1622 = Subtract(x=w2054, y=w2055) -> (x-y=w2051:dbl)
                                n1623 = Absolute Value(x=w2051) -> (abs(x)=w2050:dbl)
                                n1624 = Multiply(x=w2050, y=w2052) -> (x*y=w2057:dbl)
                                n1625 = Divide(x=w2057, y=3000.0) -> (x/y=w2053:dbl)
                                }
                                frame "High Resolution Pumping" {
                                n1626 = Subtract(x=w2063, y=w2062) -> (x-y=w2059:dbl)
                                n1627 = Absolute Value(x=w2059) -> (abs(x)=w2058:dbl)
                                n1628 = Multiply(x=w2058, y=w2061) -> (x*y=w2065:dbl)
                                n1629 = Divide(x=w2065, y=24000.0) -> (x/y=w2060:dbl)
                                }
                                }
                                n1630 = Subtract(x=w2044, y=w2043) -> (x-y=w2042:dbl)
                                n1631 = local read "Vol_now"() -> (w2040:dbl)
                                n1632 = local write "Sample Volume Diverted\ninto Column-2"(w2044) -> ()
                                n1633 = Add(x=w2042, y=w2040) -> (x+y=w2041:dbl)
                                n1634 = local write "Volume being Injected \nin this process"(w2041) -> ()
                                }
                                frame #1 {
                                n1635 = local read "Volume being Injected \nin this process"() -> (w2066:dbl)
                                n1636 = local read "Sample Volume Diverted\ninto Column-2"() -> (w2067:dbl)
                                n1637 = local write "Vol_now"(w2066) -> ()
                                n1638 = local write "Vol_previous"(w2067) -> ()
                                }
                                frame #2 {
                                n1639 = local read "Buffer-B Volume \nto be Pumped for\nSample Diversion\nto Column-2"() -> (w2069:dbl)
                                n1640 = local read "Sample Volume Diverted\ninto Column-2"() -> (w2068:dbl)
                                n1641 = local read "Stopper that ends \nthe main loops"() -> (w2070:bool)
                                n1642 = call "LSPOneStatus (SubVI).vi"("VISA Refnum in"=w2075) -> ("read buffer"=w2077:string)  [unwired: 10 in]
                                n1643 = call <vilib>:"Trim Whitespace.vi"("string"=w2077) -> ("trimmed string"=w2076:string)  [unwired: 1 in]
                                n1644 = Equal?(x=w2076, y="/0`\u0003") -> (x = y?=w2074:bool)
                                n1645 = Greater Or Equal?(x=w2068, y=w2069) -> (x >= y?=w2072:bool)
                                n1646 = Or(x=w2070, y=w2072) -> (x .or. y?=w2071:bool)
                                n1647 = Or(x=w2074, y=w2071) -> (x .or. y?=w2073:bool)
                                }
                                }
                                }
                                n1648 = local read "Stopper that ends \nthe main loops"() -> (w2029:bool)
                                n1649 = case shown="True" w2029 {
                                frame False {
                                }
                                frame True {
                                n1650 = local read "VISA Refnum in\nfor Pump"() -> (w2079:refnum<visa-resource-name>)
                                n1651 = call "HardStopCurrentProcess (SubVI).vi"("VISA Refnum in"=w2079) -> ()  [unwired: 11 in]
                                }
                                }
                                }
                                frame #1 {
                                n1652 = local read "VISA Refnum in\nfor Pump"() -> (w2081:refnum<visa-resource-name>)
                                n1653 = local write "Pause Data Collection"(TRUE ("Pause Data Collection")) -> ()
                                n1654 = call "HardStopCurrentProcess (SubVI).vi"("VISA Refnum in"=w2081) -> ()  [unwired: 11 in]
                                }
                                frame #2 {
                                n1655 = local read "VISA Refnum in\nfor Pump"() -> (w2082:refnum<visa-resource-name>)
                                n1656 = call "PortChanger (SubVI).vi"("Port Number"="1", "VISA Refnum in"=w2082) -> ()  [unwired: 10 in]
                                }
                                frame #3 {
                                n1657 = local read "VISA Refnum in\nfor Pump"() -> (w2088:refnum<visa-resource-name>)
                                n1658 = local read "Volume of Syringe"() -> (w2084:dbl)
                                n1659 = call "GoToAbsolutePosition(SubVI).vi"("Absolute Volume Position in Syringe (in ul)"=0.0, "Volume of Syringe"=w2084, "Resolution of Pumping"=T2."Standard Pumping", "Flow Rate (ul/min)"=150.0, "VISA Refnum in"=w2088) -> ()  [unwired: 6 in, 1 out]
                                }
                                frame #4 {
                                n1660 = local read "VISA Refnum in\nfor Pump"() -> (w2090:refnum<visa-resource-name>)
                                n1661 = local write "Divert Sample \ninto Column-2"(FALSE ("Divert Sample \ninto Column-2")) -> ()
                                n1662 = call "ProcessCompletionWaiter (SubVI).vi"("VISA Refnum in"=w2090) -> ()  [unwired: 11 in]
                                }
                                }
                              }
                            }
                          }
                          frame #15 {
                            # "Keeps the On-Chip Valves V1 and V3 closed"
                            # "Switch to Port-5/8"
                            # "Port-5/8 of pump is connected to Buffer-C1/C2"
                            # "Keeps the AMF valve after column-1 open and valve after column-2 closed"
                            n1663 = local read "VISA Refnum in\nfor Pump"() -> (w2103:refnum<visa-resource-name>)
                            n1664 = local write "Pause Data Collection"(TRUE ("Pause Data Collection")) -> ()
                            n1665 = Wait (ms)(milliseconds to wait=u32 500) -> ()  [unwired: 1 out]
                            n1666 = local write "Affinity On"(FALSE ("Affinity On")) -> ()
                            n1667 = local read "Port for \nC2-Elution"() -> (w2094:string)
                            n1668 = local write "Affinity Elution On"(FALSE ("Affinity Elution On")) -> ()
                            n1669 = call "PortChanger (SubVI).vi"("Port Number"=w2094, "VISA Refnum in"=w2103) -> ()  [unwired: 10 in]
                            n1670 = local read "VISA Refnum in\nfor Valve"() -> (w2097:refnum<visa-resource-name>)
                            n1671 = local read "External Valve \nCLOSED"() -> (w2096:string)
                            n1672 = local write "Valve V1 Open"(FALSE ("Valve V1 Open")) -> ()
                            n1673 = local write "Valve V2 Open"(FALSE ("Valve V2 Open")) -> ()
                            n1674 = local write "Valve V3 Open"(FALSE ("Valve V3 Open")) -> ()
                            n1675 = local write "Valve V4 Open"(FALSE ("Valve V4 Open")) -> ()
                            n1676 = call "PortChanger_Valve (SubVI).vi"("Port Number"=w2096, "VISA Refnum in"=w2097) -> ()  [unwired: 10 in]
                            n1677 = local write "Valve V5 Open"(FALSE ("Valve V5 Open")) -> ()
                            n1678 = local write "Valve V6 Open"(FALSE ("Valve V6 Open")) -> ()
                            n1679 = local write "Valve V7 Open"(FALSE ("Valve V7 Open")) -> ()
                          }
                          frame #16 {
                            n1680 = local read "VISA Refnum in\nfor Pump"() -> (w2107:refnum<visa-resource-name>)
                            n1681 = call "ProcessCompletionWaiter (SubVI).vi"("VISA Refnum in"=w2107) -> ()  [unwired: 11 in]
                            n1682 = local write "Start the Process"(FALSE ("Start the Process")) -> ()
                          }
                          frame #17 {
                            n1683 = local read "Stopper that ends \nthe main loops"() -> (w2111:bool)
                            n1684 = local read "Start the Process"() -> (w2112:bool)
                            n1685 = Or(x=w2112, y=w2111) -> (x .or. y?=w2110:bool)
                            n1686 = local write "Elution of Column-1"(FALSE ("Elution of Column-1")) -> ()
                            n1687 = case shown="False" w2110 {
                              frame False {
                                n1688 = while {
                                stop <- w2116 stop-if-true
                                n1689 = local read "Stopper that ends \nthe main loops"() -> (w2117:bool)
                                n1690 = local read "Start the Process"() -> (w2118:bool)
                                n1691 = Or(x=w2118, y=w2117) -> (x .or. y?=w2116:bool)
                                n1692 = Wait (ms)(milliseconds to wait=u32 10) -> ()  [unwired: 1 out]
                                }
                                n1693 = One Button Dialog(message="Move to Column-2 detection zone and Press 'Start the Process' Button.") -> ()  [unwired: 1 in, 1 out]
                              }
                              frame True {
                              }
                            }
                            n1694 = local write "Volume being Injected \nin this process"(0.0 ("Volume being Injected \nin this process")) -> ()
                            n1695 = local write "Elution of Column-2"(TRUE ("Elution of Column-2")) -> ()
                          }
                          frame #18 {
                            # "If Yes, it will clean the SEC buffer from port-8 tubing else it will clean the pump valve a bit"
                            n1696 = local read "Clean the \nBuffer-C2 tubing"() -> (w2119:bool)
                            n1697 = case shown="False" w2119 {
                              frame False {
                                n1698 = stacked-sequence {
                                frame #0 {
                                n1699 = local read "VISA Refnum in\nfor Pump"() -> (w2121:refnum<visa-resource-name>)
                                n1700 = local read "Port for \nC2-Elution"() -> (w2120:string)
                                n1701 = call "PortChanger (SubVI).vi"("Port Number"=w2120, "VISA Refnum in"=w2121) -> ()  [unwired: 10 in]
                                }
                                frame #1 {
                                n1702 = local read "VISA Refnum in\nfor Pump"() -> (w2122:refnum<visa-resource-name>)
                                n1703 = call "ProcessCompletionWaiter (SubVI).vi"("VISA Refnum in"=w2122) -> ()  [unwired: 11 in]
                                }
                                frame #2 {
                                n1704 = local read "Buffer-C2 Pumping\nResolution"() -> (w2125:T2)
                                n1705 = local read "VISA Refnum in\nfor Pump"() -> (w2127:refnum<visa-resource-name>)
                                n1706 = local read "V-S"() -> (w2123:dbl)
                                n1707 = local read "Volume of Syringe"() -> (w2126:dbl)
                                n1708 = call "RPickUp(SubVI).vi"("Volume to be picked up"=w2123, "Volume of Syringe"=w2126, "Resolution of PickUP"=w2125, "PickUp Flow Rate (ul/min)"=150.0, "VISA Refnum in"=w2127) -> ()  [unwired: 6 in, 1 out]
                                }
                                frame #3 {
                                n1709 = local read "Stopper that ends \nthe main loops"() -> (w2128:bool)
                                n1710 = local read "VISA Refnum in\nfor Pump"() -> (w2129:refnum<visa-resource-name>)
                                n1711 = case shown="True" w2128 {
                                frame False {
                                }
                                frame True {
                                n1712 = local read "VISA Refnum in\nfor Pump"() -> (w2130:refnum<visa-resource-name>)
                                n1713 = call "HardStopCurrentProcess (SubVI).vi"("VISA Refnum in"=w2130) -> ()  [unwired: 11 in]
                                }
                                }
                                n1714 = call "ProcessCompletionWaiter (SubVI).vi"("VISA Refnum in"=w2129) -> ()  [unwired: 11 in]
                                }
                                frame #4 {
                                n1715 = local read "VISA Refnum in\nfor Pump"() -> (w2132:refnum<visa-resource-name>)
                                n1716 = call "PortChanger (SubVI).vi"("Port Number"="1", "VISA Refnum in"=w2132) -> ()  [unwired: 10 in]
                                }
                                frame #5 {
                                n1717 = local read "Stopper that ends \nthe main loops"() -> (w2133:bool)
                                n1718 = local read "VISA Refnum in\nfor Pump"() -> (w2134:refnum<visa-resource-name>)
                                n1719 = case shown="True" w2133 {
                                frame False {
                                }
                                frame True {
                                n1720 = local read "VISA Refnum in\nfor Pump"() -> (w2135:refnum<visa-resource-name>)
                                n1721 = call "HardStopCurrentProcess (SubVI).vi"("VISA Refnum in"=w2135) -> ()  [unwired: 11 in]
                                }
                                }
                                n1722 = call "ProcessCompletionWaiter (SubVI).vi"("VISA Refnum in"=w2134) -> ()  [unwired: 11 in]
                                }
                                frame #6 {
                                n1723 = local read "VISA Refnum in\nfor Pump"() -> (w2140:refnum<visa-resource-name>)
                                n1724 = local read "Volume of Syringe"() -> (w2137:dbl)
                                n1725 = call "GoToAbsolutePosition(SubVI).vi"("Absolute Volume Position in Syringe (in ul)"=0.0, "Volume of Syringe"=w2137, "Resolution of Pumping"=T2."Standard Pumping", "Flow Rate (ul/min)"=150.0, "VISA Refnum in"=w2140) -> ()  [unwired: 6 in, 1 out]
                                }
                                frame #7 {
                                n1726 = local read "Stopper that ends \nthe main loops"() -> (w2141:bool)
                                n1727 = local read "VISA Refnum in\nfor Pump"() -> (w2142:refnum<visa-resource-name>)
                                n1728 = case shown="True" w2141 {
                                frame False {
                                }
                                frame True {
                                n1729 = local read "VISA Refnum in\nfor Pump"() -> (w2143:refnum<visa-resource-name>)
                                n1730 = call "HardStopCurrentProcess (SubVI).vi"("VISA Refnum in"=w2143) -> ()  [unwired: 11 in]
                                }
                                }
                                n1731 = call "ProcessCompletionWaiter (SubVI).vi"("VISA Refnum in"=w2142) -> ()  [unwired: 11 in]
                                }
                                }
                              }
                              frame True {
                                n1732 = for {
                                N: 2 -> [_]
                                n1733 = stacked-sequence {
                                frame #0 {
                                n1734 = local read "VISA Refnum in\nfor Pump"() -> (w2146:refnum<visa-resource-name>)
                                n1735 = local read "Port for \nC2-Elution"() -> (w2145:string)
                                n1736 = call "PortChanger (SubVI).vi"("Port Number"=w2145, "VISA Refnum in"=w2146) -> ()  [unwired: 10 in]
                                }
                                frame #1 {
                                n1737 = local read "VISA Refnum in\nfor Pump"() -> (w2147:refnum<visa-resource-name>)
                                n1738 = call "ProcessCompletionWaiter (SubVI).vi"("VISA Refnum in"=w2147) -> ()  [unwired: 11 in]
                                }
                                frame #2 {
                                n1739 = local read "Buffer-C2 Pumping\nResolution"() -> (w2150:T2)
                                n1740 = local read "VISA Refnum in\nfor Pump"() -> (w2152:refnum<visa-resource-name>)
                                n1741 = local read "Apparent Volume\nof Syringe"() -> (w2148:dbl)
                                n1742 = local read "Volume of Syringe"() -> (w2151:dbl)
                                n1743 = call "RPickUp(SubVI).vi"("Volume to be picked up"=w2148, "Volume of Syringe"=w2151, "Resolution of PickUP"=w2150, "PickUp Flow Rate (ul/min)"=150.0, "VISA Refnum in"=w2152) -> ()  [unwired: 6 in, 1 out]
                                }
                                frame #3 {
                                n1744 = local read "Stopper that ends \nthe main loops"() -> (w2153:bool)
                                n1745 = local read "VISA Refnum in\nfor Pump"() -> (w2154:refnum<visa-resource-name>)
                                n1746 = case shown="True" w2153 {
                                frame False {
                                }
                                frame True {
                                n1747 = local read "VISA Refnum in\nfor Pump"() -> (w2155:refnum<visa-resource-name>)
                                n1748 = call "HardStopCurrentProcess (SubVI).vi"("VISA Refnum in"=w2155) -> ()  [unwired: 11 in]
                                }
                                }
                                n1749 = call "ProcessCompletionWaiter (SubVI).vi"("VISA Refnum in"=w2154) -> ()  [unwired: 11 in]
                                }
